vi "Driving.vi"(11 "input cluster":T1) -> ()   [LabVIEW 2015]
uses:
  Joystick/ControlsToCommands.ctl
  References/Refnums.vi
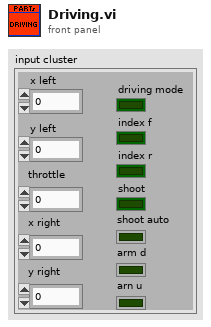
[diagram p1: front panel]
types:
  T1 = typedef "ControlsToCommands.ctl" = cluster{"x left":dbl, "y left":dbl, "throttle":dbl, "x right":dbl, "y right":dbl, "driving mode":bool, "index f":bool, "index r":bool, "shoot":bool, "shoot auto":bool, "arm d":bool, "arn u":bool}
  T2 = typedef "WPI_MotorControlDeviceRef.ctl" = cluster{"DeviceStatus":errorcluster, "Type":T3, "PWM":cluster{"PWM Channel":T4, "DeadBand":T5}, "CAN":cluster{"Device Number":u8, "Control Mode":T6, "Semaphore":T7, "Max Vout":dbl, "TalonSRX Control Mode":T8}, "Invert":bool}
  T3 = typedef "WPI_MotorControlType.ctl" = enum16{"PWM", "CAN", "CANTalonSRX"}
  T4 = typedef "FPGA_DIOPWMChannel.ctl" = enum8{"PWM 0", "PWM 1", "PWM 2", "PWM 3", "PWM 4", "PWM 5", "PWM 6", "PWM 7", "PWM 8", "PWM 9", "PWM MXP 0", "PWM MXP 1", "PWM MXP 2", "PWM MXP 3", "PWM MXP 4", "PWM MXP 5", "PWM MXP 6", "PWM MXP 7", "PWM MXP 8", "PWM MXP 9", "Invalid"}
  T5 = typedef "WPI_PWMDeadband.ctl" = cluster{"Name":string, "maxPositivePwm":i32, "minPositivePwm":i32, "centerPwm":i32, "maxNegativePwm":i32, "minNegativePwm":i32, "angularRange":u16}
  T6 = typedef "WPI_CANJaguar_ControlMode.ctl" = enum8{"Percent VBus", "Current", "Speed", "Position", "Voltage"}
  T7 = typedef "Semaphore RefNum" = refnum<k1>
  T8 = typedef "WPI_CANTalonSRX_APIControlMode.ctl" = enum8{"Percent VBus", "Speed", "Position", "Slave", "Unchanged / Invalid", "Voltage Compensation", "Current", "Motion Profile"}
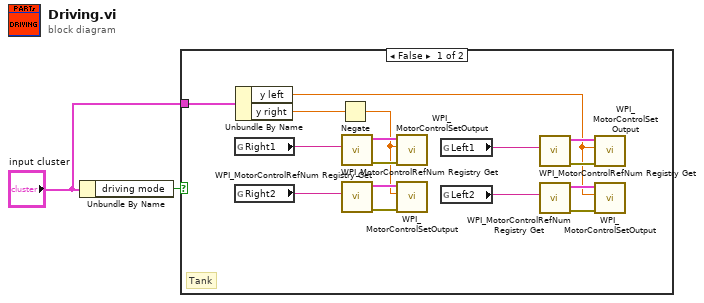
[diagram p0: block diagram]
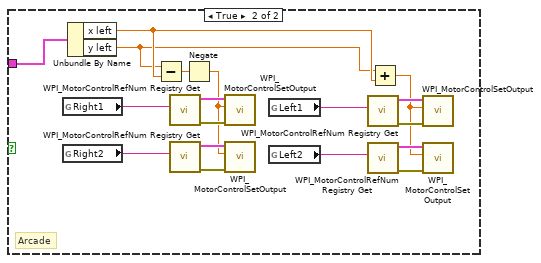
[diagram p2: hidden frame]
diagram:
  n1 = Unbundle By Name("input cluster") -> ("driving mode"=w2:bool)
  n2 = case shown="False" w2 {
    tunnel: "input cluster" -> [w5 w23]
    frame False {
      # "Tank"
      n3 = global read "Refnums.vi" "Right1"() -> (w10:string)
      n4 = global read "Refnums.vi" "Right2"() -> (w9:string)
      n5 = Unbundle By Name(w5) -> ("y left"=w3:dbl, "y right"=w4:dbl)
      n6 = Negate(x=w4) -> (-x=w6:dbl)
      n7 = call <vilib>:"WPI_MotorControlRefNum Registry Get.vi"("refnum name"=w10) -> ("error out"=w12:errorcluster, "MotorControlDevRef"=w11:T2)  [unwired: 9 in]
      n8 = call <vilib>:"WPI_MotorControlRefNum Registry Get.vi"("refnum name"=w9) -> ("error out"=w7:errorcluster, "MotorControlDevRef"=w8:T2)  [unwired: 9 in]
      n9 = call <vilib>:"WPI_MotorControlSetOutput.vi"("error in (no error)"=w12, "Output"=w6, "MotorControlDevRef"=w11) -> ()  [unwired: 6 in, 3 out]
      n10 = call <vilib>:"WPI_MotorControlSetOutput.vi"("error in (no error)"=w7, "Output"=w6, "MotorControlDevRef"=w8) -> ()  [unwired: 6 in, 3 out]
      n11 = global read "Refnums.vi" "Left1"() -> (w13:string)
      n12 = global read "Refnums.vi" "Left2"() -> (w16:string)
      n13 = call <vilib>:"WPI_MotorControlRefNum Registry Get.vi"("refnum name"=w13) -> ("error out"=w15:errorcluster, "MotorControlDevRef"=w14:T2)  [unwired: 9 in]
      n14 = call <vilib>:"WPI_MotorControlRefNum Registry Get.vi"("refnum name"=w16) -> ("error out"=w18:errorcluster, "MotorControlDevRef"=w17:T2)  [unwired: 9 in]
      n15 = call <vilib>:"WPI_MotorControlSetOutput.vi"("error in (no error)"=w15, "Output"=w3, "MotorControlDevRef"=w14) -> ()  [unwired: 6 in, 3 out]
      n16 = call <vilib>:"WPI_MotorControlSetOutput.vi"("error in (no error)"=w18, "Output"=w3, "MotorControlDevRef"=w17) -> ()  [unwired: 6 in, 3 out]
    }
    frame True {
      # "Arcade"
      n17 = global read "Refnums.vi" "Right1"() -> (w28:string)
      n18 = global read "Refnums.vi" "Right2"() -> (w27:string)
      n19 = Unbundle By Name(w23) -> ("x left"=w20:dbl, "y left"=w19:dbl)
      n20 = Subtract(x=w19, y=w20) -> (x-y=w22:dbl)
      n21 = call <vilib>:"WPI_MotorControlRefNum Registry Get.vi"("refnum name"=w28) -> ("error out"=w30:errorcluster, "MotorControlDevRef"=w29:T2)  [unwired: 9 in]
      n22 = call <vilib>:"WPI_MotorControlRefNum Registry Get.vi"("refnum name"=w27) -> ("error out"=w25:errorcluster, "MotorControlDevRef"=w26:T2)  [unwired: 9 in]
      n23 = Negate(x=w22) -> (-x=w24:dbl)
      n24 = call <vilib>:"WPI_MotorControlSetOutput.vi"("error in (no error)"=w30, "Output"=w24, "MotorControlDevRef"=w29) -> ()  [unwired: 6 in, 3 out]
      n25 = call <vilib>:"WPI_MotorControlSetOutput.vi"("error in (no error)"=w25, "Output"=w24, "MotorControlDevRef"=w26) -> ()  [unwired: 6 in, 3 out]
      n26 = global read "Refnums.vi" "Left1"() -> (w31:string)
      n27 = global read "Refnums.vi" "Left2"() -> (w34:string)
      n28 = call <vilib>:"WPI_MotorControlRefNum Registry Get.vi"("refnum name"=w31) -> ("error out"=w33:errorcluster, "MotorControlDevRef"=w32:T2)  [unwired: 9 in]
      n29 = call <vilib>:"WPI_MotorControlRefNum Registry Get.vi"("refnum name"=w34) -> ("error out"=w36:errorcluster, "MotorControlDevRef"=w35:T2)  [unwired: 9 in]
      n30 = Add(x=w19, y=w20) -> (x+y=w21:dbl)
      n31 = call <vilib>:"WPI_MotorControlSetOutput.vi"("error in (no error)"=w33, "Output"=w21, "MotorControlDevRef"=w32) -> ()  [unwired: 6 in, 3 out]
      n32 = call <vilib>:"WPI_MotorControlSetOutput.vi"("error in (no error)"=w36, "Output"=w21, "MotorControlDevRef"=w35) -> ()  [unwired: 6 in, 3 out]
    }
  }
